vi "gfitsio-movabs-hdu.vi"(7 "hdunum":i32, 8 "error in (no error)":errorcluster, 11 "gfits refnum":T2) -> (0 "error out":errorcluster, 2 "hdutype":T1 items=["ANY_HDU"=-1, "IMAGE_HDU"=0, "ASCII_TBL"=1, "BINARY_TBL"=2], 3 "dup gfits refnum":T2)   [LabVIEW 2019, in "gfitsio.lvlib"]
doc: "Move to a different HDU in the file specified by the absolute HDU number (starting with 1 for the primary array) in the FITS file. <B>hdutype</B> contains the type of the new current HDU."
uses:
  gfitsio.lvlib
  gfitsio-refnum.ctl
  cfitsio-hdutypes.ctl
  gfitsio.dll
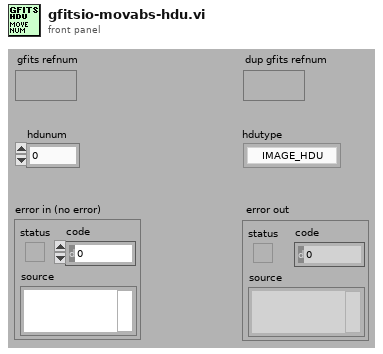
[diagram p1: front panel]
types:
  T1 = typedef "gfitsio.lvlib/cfitsio-hdutypes.ctl" = i32
  T2 = typedef "gfitsio.lvlib/gfitsio-refnum.ctl" = refnum<k1>
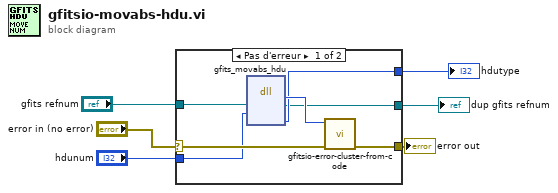
[diagram p0: block diagram]
diagram:
  n1 = case shown="Pas d'erreur" "error in (no error)" {
    selector: "error in (no error)" -> [w12 w15]
    tunnel: [w11 w15] -> w6
    tunnel: "hdunum" -> [w9 _]
    tunnel: [w8 w14] -> w3
    tunnel: "gfits refnum" -> [w7 w14]
    tunnel: [w10 _] -> w1
    frame No Error {
      n2 = dll-call lib="C:/BonOMM_git/SubVIs/gfitsio/gfitsio.dll" fn="gfits_movabs_hdu"("gfits refnum"=w7, "hdunum"=w9) -> (w13:i32, "gfits refnum"=w8:T2, "hdutype"=w10:i32)  [unwired: 5 in, 2 out]
      n3 = call "gfitsio-error-cluster-from-code.vi"("error in (no error)"=w12, "error code"=w13) -> ("error out"=w11:errorcluster)  [unwired: 9 in]
    }
    frame Error {
    }
  }
  "error out" <- w6
  "dup gfits refnum" <- w3
  "hdutype" <- w1
